vi "rohitBoolean.vi"() -> ()   [LabVIEW 2009]
panel:
  in  "Input B":bool
  out "Output":bool
  in  "Input A":bool
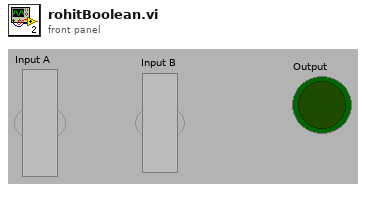
[diagram p1: front panel]
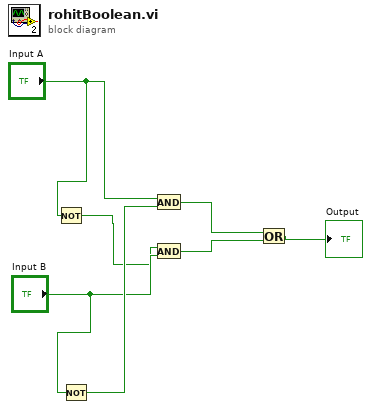
[diagram p0: block diagram]
diagram:
  n1 = Not(x="Input A") -> (.not. x?=w1:bool)
  n2 = Not(x="Input B") -> (.not. x?=w6:bool)
  n3 = And(x="Input A", y=w6) -> (x .and. y?=w4:bool)
  n4 = And(x=w1, y="Input B") -> (x .and. y?=w3:bool)
  n5 = Or(x=w4, y=w3) -> (x .or. y?=→"Output":bool)
